vi "Config Core.vi"(8 "Error In":errorcluster, 10 "FileConfig In":refnum<class "FileConfig.lvclass">, 11 "Hardware In":refnum<class "ILogger.lvclass">) -> (0 "Error Out":errorcluster, 2 "FileConfig Out":refnum<class "FileConfig.lvclass">, 3 "Hardware Out":refnum<class "ILogger.lvclass">)   [LabVIEW 2020, in "FileConfig.lvclass"]
uses:
  FileConfig.lvclass
  FileLogger/FileLogger.lvclass
  C:/Repo/LabVIEW-SOLID-Examples/Template-Logger/FileLogger/FileLogger.lvclass
  C:/Repo/LabVIEW-SOLID-Examples/Template-Logger/ILogger/ILogger.lvclass
  ILogger/ILogger.lvclass
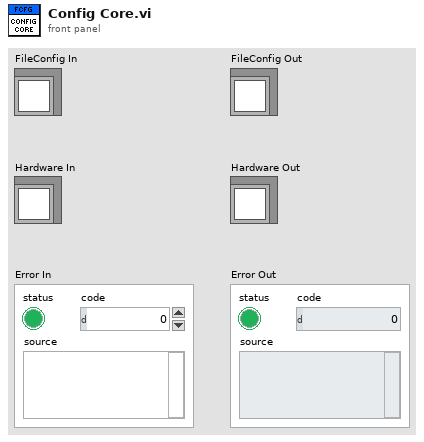
[diagram p1: front panel]
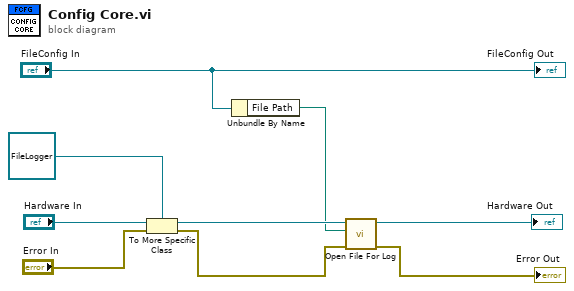
[diagram p0: block diagram]
diagram:
  n1 = To More Specific Class(target class=refnum<class "FileLogger.lvclass"> refnum ("FileLogger.lvclass"), reference="Hardware In", error in="Error In") -> (specific class reference=w6:refnum<class "FileLogger.lvclass">, error out=w4:errorcluster)
  n2 = Unbundle By Name("FileConfig In") -> ("File Path"=w1:path)
  n3 = call "Open File For Log.vi"("Error In"=w4, "File Path"=w1, "FileLogger In"=w6) -> ("Error Out"=→"Error Out":errorcluster, "FileLogger Out"=→"Hardware Out":refnum<class "FileLogger.lvclass">)  [unwired: 7 in]
  "FileConfig Out" <- "FileConfig In"
